vi "set_multiplexor.vi"(3 "error in (no error)":errorcluster, 4 "Common Input Channel":u16, 5 "Pixel Input Channel":u16) -> (0 "error out":errorcluster)   [LabVIEW 2016]
uses:
  C:/Program Files (x86)/National Instruments/LabVIEW 2016/instr.lib/QuickMux/QuickMux.lvlib
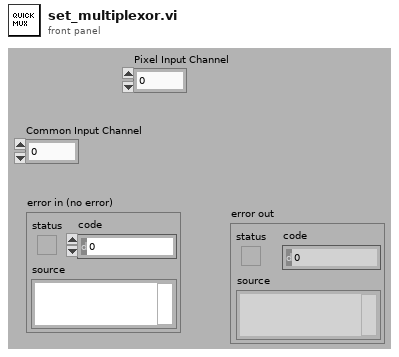
[diagram p1: front panel]
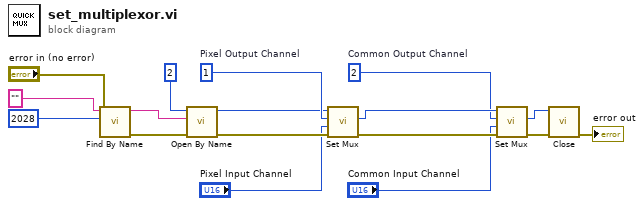
[diagram p0: block diagram]
diagram:
  w5 = u16 2  # Common Output Channel
  w12 = u16 1  # Pixel Output Channel
  n1 = call "Find By Name.vi"("error in (no error)"="error in (no error)", "length"=u16 2028, "nameList"="") -> ("error out"=w14:errorcluster, "nameList out"=w15:string)  [unwired: 5 in, 2 out]
  n2 = call "Open By Name.vi"("error in (no error)"=w14, "deviceName"=w15, "handle 2"=u64 2) -> ("error out"=w10:errorcluster, "handle"=w11:u64)  [unwired: 6 in, 1 out]
  n3 = call "Set Mux.vi"("error in (no error)"=w10, "inputChannel"="Pixel Input Channel", "outputChannel"=w12, "handle"=w11) -> ("error out"=w6:errorcluster, "handle Out"=w7:u8)  [unwired: 5 in, 1 out]
  n4 = call "Set Mux.vi"("error in (no error)"=w6, "inputChannel"="Common Input Channel", "outputChannel"=w5, "handle"=w7) -> ("error out"=w2:errorcluster, "handle Out"=w3:u8)  [unwired: 5 in, 1 out]
  n5 = call "Close.vi"("error in (no error)"=w2, "handle"=w3) -> ("error out"=→"error out":errorcluster)  [unwired: 8 in, 1 out]
